vi "Offset.vi"(10 "Point":T1, 11 "Bounds In":T2) -> (3 "Bounds Out":T2)   [LabVIEW 2019, in "2D.lvlib"]
doc: "Add a horizontal and vertical offset to the given bounds, retaining the bounds size."
uses:
  2D.lvlib
  <vilib>/Utility/miscctls.llb/LVRectTypeDef.ctl
  Point.ctl
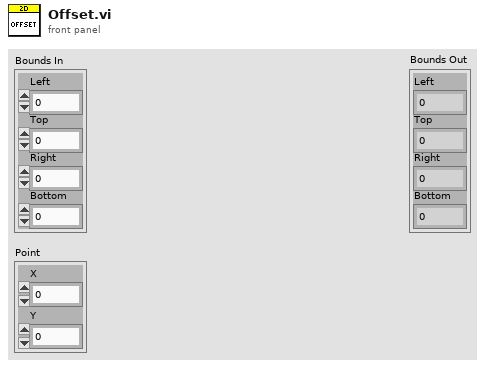
[diagram p1: front panel]
types:
  T1 = typedef "2D.lvlib/Point.ctl" = cluster{"X":i16, "Y":i16}
  T2 = typedef "LVRectTypeDef.ctl" = cluster{"Left":i16, "Top":i16, "Right":i16, "Bottom":i16}
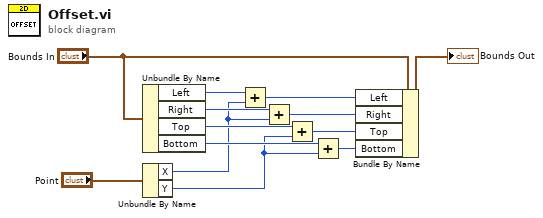
[diagram p0: block diagram]
diagram:
  n1 = Unbundle By Name("Bounds In") -> ("Left"=w12:i16, "Right"=w11:i16, "Top"=w10:i16, "Bottom"=w9:i16)
  n2 = Unbundle By Name("Point") -> ("X"=w2:i16, "Y"=w1:i16)
  n3 = Add(x=w12, y=w2) -> (x+y=w8:i16)
  n4 = Add(x=w11, y=w2) -> (x+y=w7:i16)
  n5 = Add(x=w10, y=w1) -> (x+y=w6:i16)
  n6 = Add(x=w9, y=w1) -> (x+y=w5:i16)
  n7 = Bundle By Name(cluster="Bounds In", "Left"=w8, "Right"=w7, "Top"=w6, "Bottom"=w5) -> (→"Bounds Out":T2)
